vi "Pre Launch Init.vi"(11 "Display Console in":refnum<class "Display Console.lvclass">) -> (0 "error out":errorcluster, 3 "Display Console out":refnum<class "Display Console.lvclass">)   [LabVIEW 2019, in "Display Console Actor.lvlib" / "Display Console.lvclass"]
doc: "(<B>Filename</B>: Actor Framework.lvlib:Actor.lvclass:Pre Launch Init.vi)\n\nDefines behavior that occurs after the Launch Nested Actor method is invoked but before the actor's Actor Core method begins running.\n\nBy default, this method does nothing. A descendant class may override it to define behavior."
uses:
  Display Console.lvclass
  Display Console.lvclass/Display Console.ctl
  Abstract Display Console Actor/Abstract Display Console Actor/Abstract Display Console.lvclass
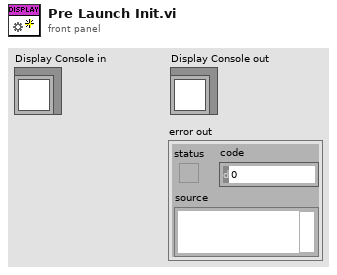
[diagram p1: front panel]
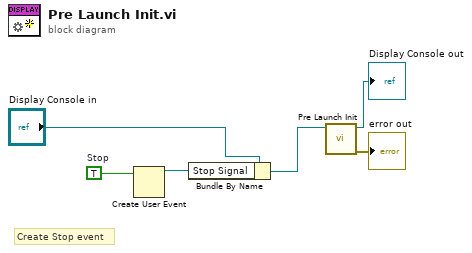
[diagram p0: block diagram]
diagram:
  w4 = TRUE  # Stop
  # "Create Stop event"
  n1 = Create User Event(user event datatype=w4) -> (user event=w3:refnum<user-event>)  [unwired: 1 in, 1 out]
  n2 = Bundle By Name(cluster="Display Console in", "Stop Signal"=w3) -> (w1:refnum<class "Display Console.lvclass">)
  n3 = call-parent "Pre Launch Init.vi"("Actor in"=w1) -> ("error out"=→"error out":errorcluster, "Actor out"=→"Display Console out":refnum<class "Display Console.lvclass">)  [unwired: 9 in]
